vi "WriteResultPathRequest.vi"(8 "error in (no error)":errorcluster, 10 "ResultPath":path, 11 "ModuleID":i32) -> (0 "error out":errorcluster)   [LabVIEW 2014, in "AnalysisPlugins.lvlib" / "AnalysisPluginsBase.lvclass"]
uses:
  AnalysisPluginsBase.lvclass
  AnalysisModule/Protected/clEventType.ctl
  <vilib>/Utility/error.llb/Error Cluster From Error Code.vi
  <vilib>/ErrorRing/Error Ring.xnode
  AnalysisModule/AnalysisModule.lvlib
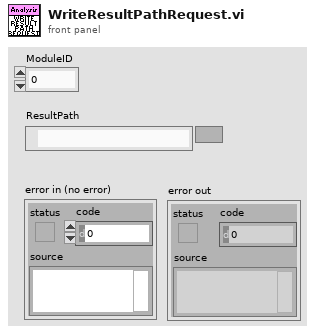
[diagram p1: front panel]
types:
  T1 = typedef "AnalysisModule.lvlib/clRequestEvents.ctl" = cluster{"StopRequest":refnum<user-event>, "PathToINI":refnum<user-event>, " LoadPlugin":refnum<user-event>, "ShowPanel":refnum<user-event>, "WriteSamples":refnum<user-event>, "ReadConfig":refnum<user-event>, "WriteConfig":refnum<user-event>, "WriteSignalParams":refnum<user-event>, "WriteTestType":refnum<user-event>, "WriteFileName":refnum<user-event>, "WriteMagCorr":refnum<user-event>, "WriteDlyCorr":refnum<user-event>, "ConfigDlg":refnum<user-event>, "WriteSensorData":refnum<user-event>, "Initialize":refnum<user-event>, "Abort":refnum<user-event>, "WriteResultPath":refnum<user-event>}
  T2 = typedef "AnalysisModule.lvlib/clEventType.ctl" = cluster{"ModuleID":i32, "Data":variant}
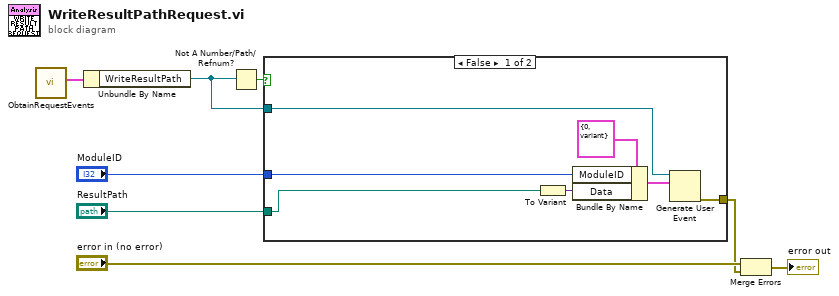
[diagram p0: block diagram]
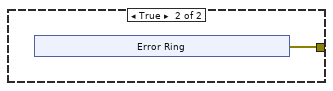
[diagram p2: hidden frame]
diagram:
  n1 = call "ObtainRequestEvents.vi"() -> ("AnalysisRequestEvents"=w8:T1)  [unwired: 10 in, 1 out]
  n2 = Unbundle By Name(w8) -> ("WriteResultPath"=w6:refnum<user-event>)
  n3 = Not A Number/Path/Refnum?(number/path/refnum=w6) -> (NaN/Path/Refnum?=w7:bool)
  n4 = case shown="False" w7 {
    tunnel: w6 -> [w11 _]
    tunnel: "ModuleID" -> [w14 _]
    tunnel: [w10 w16] -> w2
    tunnel: "ResultPath" -> [w9 _]
    frame False {
      n5 = To Variant(anything=w9) -> (Variant=w13:variant)
      n6 = Bundle By Name(cluster=T2 {"ModuleID"=0, "Data"=variant} ("clEventType"), "ModuleID"=w14, "Data"=w13) -> (w12:T2)
      n7 = Generate User Event(user event=w11, event data cluster=w12) -> (error out=w10:errorcluster)  [unwired: 2 in, 1 out]
    }
    frame True {
      n8 = xnode "Error Ring"() -> ("error out"=w16:errorcluster)
    }
  }
  n9 = Merge Errors("error in (no error)", w2) -> (→"error out":errorcluster)
